vi "题目4.vi"() -> ()   [LabVIEW 2017]
uses:
  <vilib>/measure/NI_MABase.lvlib
panel:
  in  "布尔":bool
  out "波形图":waveform(dbl)(graph)
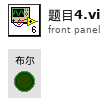
[diagram p1: front panel]
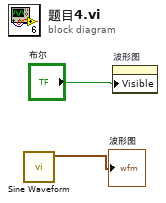
[diagram p0: block diagram]
diagram:
  n1 = call <vilib>:"Sine Waveform.vi"() -> ("signal out"=→"波形图":waveform(dbl))  [unwired: 10 in, 1 out]
  n2 = property on="波形图" class="WFGraph (严格)"("Visible"="布尔") -> ()  [unwired: 2 in, 2 out]
